vi "diff1Darray.vi"(11 "Input":dbl[](array[numeric])) -> (3 "Diff":dbl[](array[numeric]))   [LabVIEW 2016]
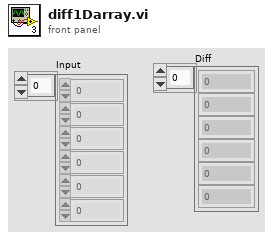
[diagram p1: front panel]
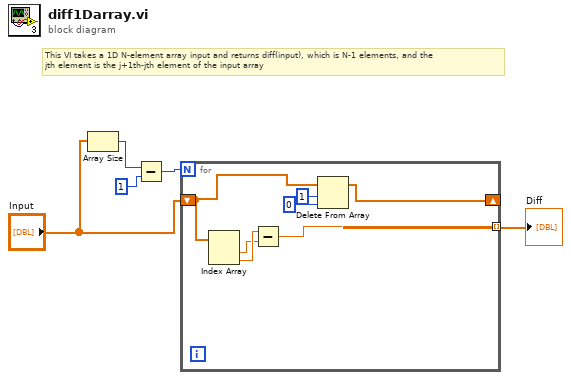
[diagram p0: block diagram]
diagram:
  # "This VI takes a 1D N-element array input and returns diff(input), which is N-1 elements, and the\njth element is the j+1th-jth element of the input array"
  n1 = Array Size(array="Input") -> (size(s)=w3:i32)
  n2 = Subtract(x=w3, y=1) -> (x-y=w1:i32)
  n3 = for {
    N: w1 -> [_]
    tunnel: [w10] -> w5 mode=indexing
    shift-right: [w6] -> _
    shift-left: "Input" -> [w9]
    n4 = Index Array(array=w9) -> (element #1=w11:dbl, element #2=w12:dbl)  [unwired: 2 in]
    n5 = Subtract(x=w12, y=w11) -> (x-y=w10:dbl)
    n6 = Delete From Array(array=w9, length=1, index=0) -> (array with subset deleted=w6:dbl[])  [unwired: 1 out]
  }
  "Diff" <- w5
